vi "MAT Save-Read Example.vi"() -> ()   [LabVIEW 2013, in "varilib.lvlib"]
uses:
  varilib.lvlib
panel:
  out "m CSG 2":string
  out "m CDB 2":string
  out "m U8 2":string
  out "m U16 2":string
  out "m I16 2":string
  out "m I32 2":string
  out "m SGL 2":string
  out "m DBL 2":string
  out "m STR 2":string
  out "CSG 2":csg[][](array[numeric]) format="%.2f"
  out "CDB 2":cdb[][](array[numeric]) format="%.2f"
  out "U8 2":u8[][](array[numeric])
  out "U16 2":u16[][](array[numeric])
  out "I16 2":i16[][](array[numeric])
  out "I32 2":i32[][](array[numeric])
  out "SGL 2":sgl[][](array[numeric]) format="%.2f"
  out "DBL 2":dbl[][](array[numeric]) format="%.2f"
  out "STR 2":string[](array[string])
  in  "Action":enum16{"save", "read"}(ring)
  in  "m CSG":string="csg"
  in  "m CDB":string="cdb"
  in  "m U8":string="u8"
  in  "m U16":string="u16"
  in  "m I16":string="i16"
  in  "m I32":string="i32"
  in  "m SGL":string="sgl"
  in  "m DBL":string="dbl"
  in  "m STR":string="str"
  in  "CSG":csg[][](array[numeric])=[[3.33+3.44i, 4.33+4.44i, 5.33+5.44i], [6.33+6.44i, 7.33+7.44i, 8.33+8.44i]] format="%.2f"
  in  "CDB":cdb[][](array[numeric])=[[1.11+2.21i, 1.12+2.22i, 1.15+2.25i], [1.16+2.26i, 1.17+2.27i, 1.18+2.28i]] format="%.2f"
  in  "U8":u8[][](array[numeric])=[[210, 211, 212], [213, 214, 215]]
  in  "U16":u16[][](array[numeric])=[[41, 42, 43], [44, 45, 46]]
  in  "I16":i16[][](array[numeric])=[[21, 22, 23], [24, 25, 26]]
  in  "I32":i32[][](array[numeric])=[[33, 34, 35], [36, 37, 38]]
  in  "SGL":sgl[][](array[numeric])=[[11.1, 12.2, 13.3], [14.4, 15.5, 16.6]] format="%.2f"
  in  "DBL":dbl[][](array[numeric])=[[1.1, 2.2, 3.3], [4.4, 5.5, 6.6]] format="%.2f"
  in  "STR":string[](array[string])=["test1", "test333"]
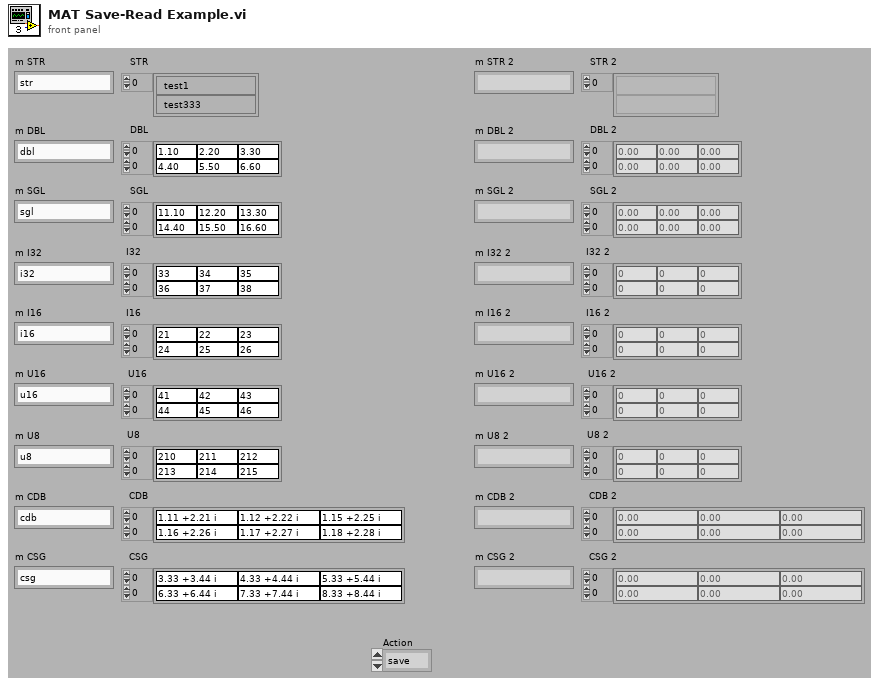
[diagram p1: front panel]
types:
  T1 = enum16{"open", "open or create", "create or replace", "create", "open (read only)"}
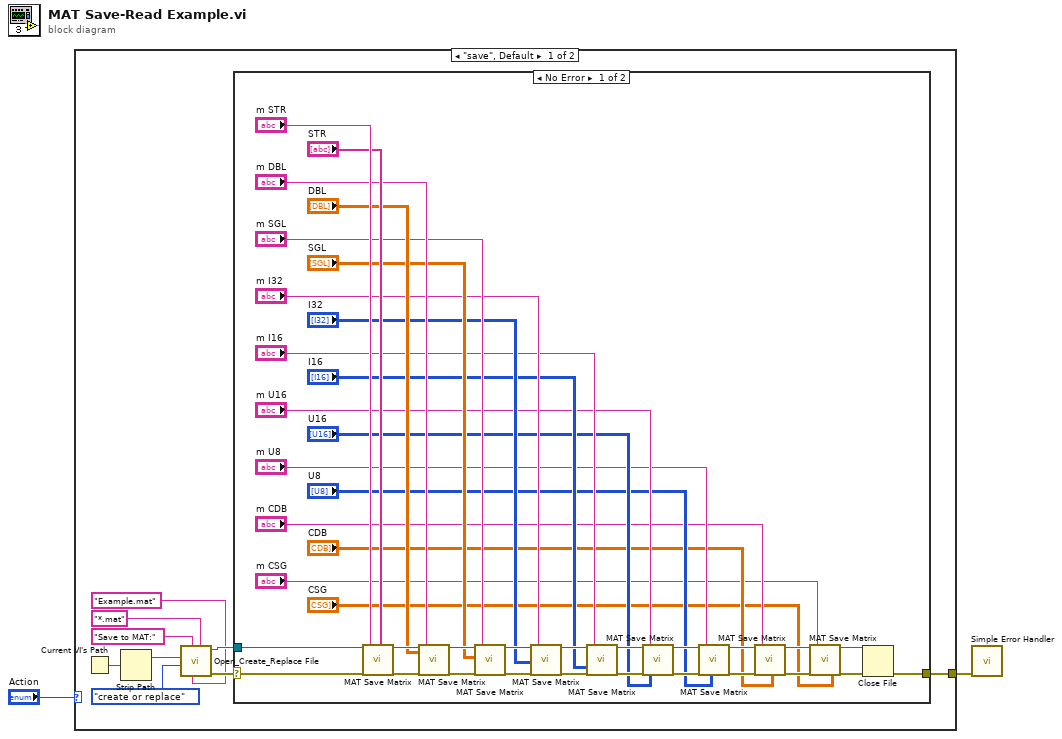
[diagram p0: block diagram]
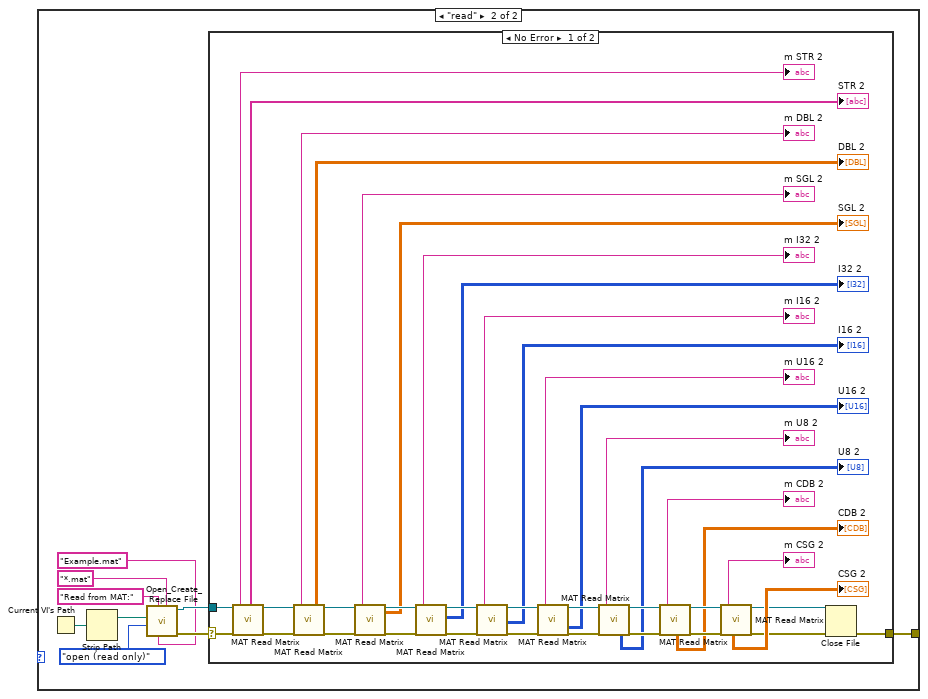
[diagram p3: hidden frame]
diagram:
  n1 = case shown="\"save\", Default" "Action" {
    tunnel: [w5 w53] -> w1
    frame "save", Default {
      n2 = Current VI's Path() -> (path=w11:path)
      n3 = Strip Path(path=w11) -> (stripped path=w10:path)  [unwired: 1 out]
      n4 = call <vilib>:"Open_Create_Replace File.vi"("pattern"="*.mat", "default name"="Example.mat" ("pattern"), "prompt"="Save to MAT:", "function (open:0)"=T1."create or replace", "start path  (Not A Path)"=w10) -> ("error out"=w7:errorcluster, "refnum"=w6:refnum<file>)  [unwired: 3 in, 2 out]
      n5 = case shown="No Error" w7 {
        selector: w7 -> [w50 w51]
        tunnel: w6 -> [w49 _]
        tunnel: [w30 w51] -> w5
        frame No Error {
          n6 = call "MAT Save Matrix.vi"("Ref Num"=w49, "error in"=w50, "Matrix Name"="m STR", "STR"="STR") -> ("Dup Ref Num"=w48:refnum<file>, "error out"=w42:errorcluster)  [unwired: 14 in]
          n7 = call "MAT Save Matrix.vi"("Ref Num"=w48, "DBL"="DBL", "error in"=w42, "Matrix Name"="m DBL") -> ("Dup Ref Num"=w36:refnum<file>, "error out"=w35:errorcluster)  [unwired: 14 in]
          n8 = call "MAT Save Matrix.vi"("Ref Num"=w36, "SGL"="SGL", "error in"=w35, "Matrix Name"="m SGL") -> ("Dup Ref Num"=w47:refnum<file>, "error out"=w41:errorcluster)  [unwired: 14 in]
          n9 = call "MAT Save Matrix.vi"("Ref Num"=w47, "I32"="I32", "error in"=w41, "Matrix Name"="m I32") -> ("Dup Ref Num"=w46:refnum<file>, "error out"=w40:errorcluster)  [unwired: 14 in]
          n10 = call "MAT Save Matrix.vi"("Ref Num"=w46, "I16"="I16", "error in"=w40, "Matrix Name"="m I16") -> ("Dup Ref Num"=w45:refnum<file>, "error out"=w39:errorcluster)  [unwired: 14 in]
          n11 = call "MAT Save Matrix.vi"("Ref Num"=w45, "error in"=w39, "Matrix Name"="m U16", "U16"="U16") -> ("Dup Ref Num"=w44:refnum<file>, "error out"=w38:errorcluster)  [unwired: 14 in]
          n12 = call "MAT Save Matrix.vi"("Ref Num"=w44, "error in"=w38, "Matrix Name"="m U8", "U8"="U8") -> ("Dup Ref Num"=w43:refnum<file>, "error out"=w37:errorcluster)  [unwired: 14 in]
          n13 = call "MAT Save Matrix.vi"("Ref Num"=w43, "error in"=w37, "Matrix Name"="m CDB", "CDB"="CDB") -> ("Dup Ref Num"=w34:refnum<file>, "error out"=w33:errorcluster)  [unwired: 14 in]
          n14 = call "MAT Save Matrix.vi"("Ref Num"=w34, "error in"=w33, "Matrix Name"="m CSG", "CSG"="CSG") -> ("Dup Ref Num"=w32:refnum<file>, "error out"=w31:errorcluster)  [unwired: 14 in]
          n15 = Close File(refnum=w32, error in=w31) -> (error out=w30:errorcluster)  [unwired: 1 out]
        }
        frame Error {
        }
      }
    }
    frame "read" {
      n16 = Current VI's Path() -> (path=w60:path)
      n17 = Strip Path(path=w60) -> (stripped path=w59:path)  [unwired: 1 out]
      n18 = call <vilib>:"Open_Create_Replace File.vi"("pattern"="*.mat", "default name"="Example.mat" ("pattern"), "prompt"="Read from MAT:", "function (open:0)"=T1."open (read only)", "start path  (Not A Path)"=w59) -> ("error out"=w55:errorcluster, "refnum"=w54:refnum<file>)  [unwired: 3 in, 2 out]
      n19 = case shown="No Error" w55 {
        selector: w55 -> [w97 w100]
        tunnel: w54 -> [w98 _]
        tunnel: [w99 w100] -> w53
        frame No Error {
          n20 = call "MAT Read Matrix.vi"("Ref Num"=w98, "Error In"=w97) -> ("Matrix Name"=→"m STR 2":string, "STR"=→"STR 2":string[], "Dup Ref Num"=w93:refnum<file>, "error out"=w94:errorcluster)  [unwired: 5 in, 9 out]
          n21 = call "MAT Read Matrix.vi"("Ref Num"=w93, "Error In"=w94) -> ("Matrix Name"=→"m DBL 2":string, "DBL"=→"DBL 2":dbl[][], "Dup Ref Num"=w96:refnum<file>, "error out"=w95:errorcluster)  [unwired: 5 in, 9 out]
          n22 = call "MAT Read Matrix.vi"("Ref Num"=w96, "Error In"=w95) -> ("Matrix Name"=→"m SGL 2":string, "Dup Ref Num"=w92:refnum<file>, "SGL"=→"SGL 2":sgl[][], "error out"=w91:errorcluster)  [unwired: 5 in, 9 out]
          n23 = call "MAT Read Matrix.vi"("Ref Num"=w92, "Error In"=w91) -> ("Matrix Name"=→"m I32 2":string, "Dup Ref Num"=w88:refnum<file>, "I32"=→"I32 2":i32[][], "error out"=w84:errorcluster)  [unwired: 5 in, 9 out]
          n24 = call "MAT Read Matrix.vi"("Ref Num"=w88, "Error In"=w84) -> ("Matrix Name"=→"m I16 2":string, "Dup Ref Num"=w87:refnum<file>, "I16"=→"I16 2":i16[][], "error out"=w83:errorcluster)  [unwired: 5 in, 9 out]
          n25 = call "MAT Read Matrix.vi"("Ref Num"=w87, "Error In"=w83) -> ("Matrix Name"=→"m U16 2":string, "Dup Ref Num"=w90:refnum<file>, "U16"=→"U16 2":u16[][], "error out"=w89:errorcluster)  [unwired: 5 in, 9 out]
          n26 = call "MAT Read Matrix.vi"("Ref Num"=w90, "Error In"=w89) -> ("Matrix Name"=→"m U8 2":string, "U8"=→"U8 2":u8[][], "Dup Ref Num"=w86:refnum<file>, "error out"=w82:errorcluster)  [unwired: 5 in, 9 out]
          n27 = call "MAT Read Matrix.vi"("Ref Num"=w86, "Error In"=w82) -> ("Matrix Name"=→"m CDB 2":string, "CDB"=→"CDB 2":cdb[][], "Dup Ref Num"=w85:refnum<file>, "error out"=w81:errorcluster)  [unwired: 5 in, 9 out]
          n28 = call "MAT Read Matrix.vi"("Ref Num"=w85, "Error In"=w81) -> ("Matrix Name"=→"m CSG 2":string, "CSG"=→"CSG 2":csg[][], "Dup Ref Num"=w62:refnum<file>, "error out"=w61:errorcluster)  [unwired: 5 in, 9 out]
          n29 = Close File(refnum=w62, error in=w61) -> (error out=w99:errorcluster)  [unwired: 1 out]
        }
        frame Error {
        }
      }
    }
  }
  n30 = call <vilib>:"Simple Error Handler.vi"("error in (no error)"=w1) -> ()  [unwired: 4 in, 5 out]
